vi "FTW-Reflection-Array.vi"(7 "Array":variant) -> (8 "Default Array Element":variant, 10 "Number of Dimensions":i32)   [LabVIEW 2014]
panel:
  # "Inputs"
  # "Outputs"
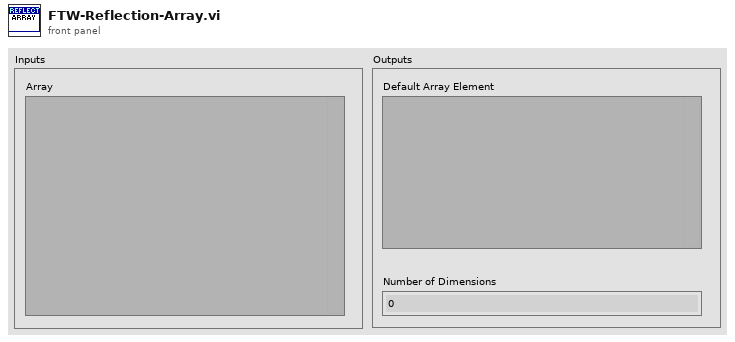
[diagram p1: front panel]
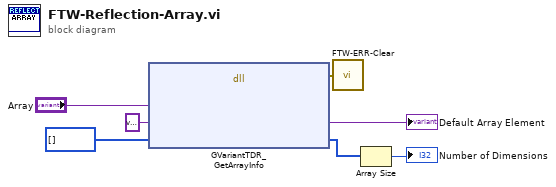
[diagram p0: block diagram]
diagram:
  n1 = dll-call lib="LabVIEW" fn="GVariantTDR_GetArrayInfo"("Array as a Variant"="Array", "Default Array Element"=variant, "Dimensions"=i32[] []) -> (error out=w5:errorcluster, "Default Array Element"=→"Default Array Element":variant, "Dimensions"=w3:i32[])  [unwired: 5 in, 1 out]
  n2 = call "FTW-ERR-Clear.vi"("error to snuff"=w5) -> ()  [unwired: 1 out]
  n3 = Array Size(array=w3) -> (size(s)=→"Number of Dimensions":i32)
